vi "Apply Speed.vi"(8 "error in (no error)":errorcluster, 11 "Tool Funnel in":refnum<class "Tool Funnel.lvclass">) -> (0 "error out":errorcluster, 3 "Tool Funnel out":refnum<class "Tool Funnel.lvclass">)   [LabVIEW 2019, in "Tool Funnel.lvclass"]
uses:
  Tool Funnel.lvclass
  Settings/ObjectSettings/ObjectSettings.lvclass/ObjectSettings.ctl
  Settings/Funnel Settings/Funnel Settings.lvclass
  C:/Users/Albro/Documents/GitHub/AFM-Lithography/lvsrc/Classes/Settings/ObjectSettings/ObjectSettings.lvclass
  Settings/ObjectSettings/ObjectSettings.lvclass
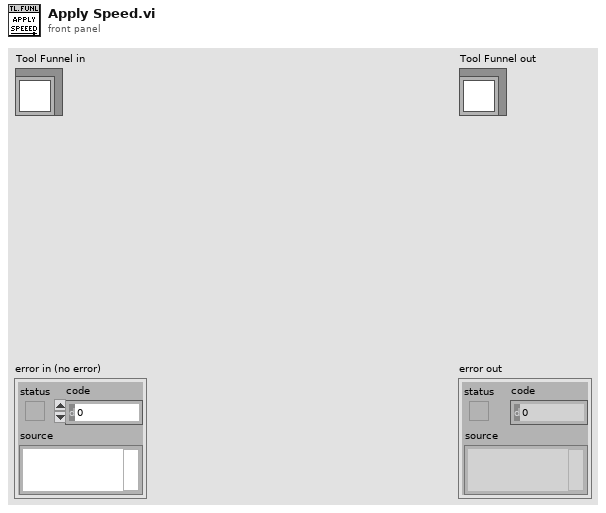
[diagram p1: front panel]
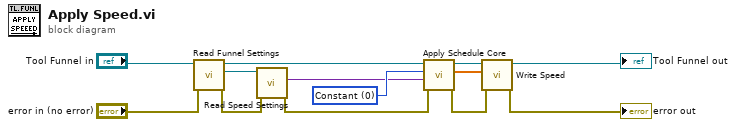
[diagram p0: block diagram]
diagram:
  w13 = u16 0 items=["Constant", "Ramp", "Function", "Formula"] ("Schedule")
  n1 = call-dynamic "Read Funnel Settings.vi"("error in (no error)"="error in (no error)", "Tool Funnel in"="Tool Funnel in") -> ("error out"=w2:errorcluster, "Funnel Settings.lvclass"=w3:refnum<class "Funnel Settings.lvclass">, "Tool Funnel out"=w4:refnum<class "Tool Funnel.lvclass">)  [unwired: 7 in]
  n2 = call "Read Speed Settings.vi"("error in (no error)"=w2, "ObjectSettings in"=w3) -> ("error out"=w9:errorcluster, "Settings"=w11:variant)  [unwired: 7 in, 1 out]
  n3 = call-dynamic "Apply Schedule Core.vi"("error in (no error)"=w9, "Settings"=w11, "Schedule"=w13, "Tool Object in"=w4) -> ("error out"=w10:errorcluster, "Schedule Array"=w8:dbl[], "Tool Object out"=w12:refnum<class "Tool Funnel.lvclass">)  [unwired: 5 in]
  n4 = call-dynamic "Write Speed.vi"("error in (no error)"=w10, "Speed"=w8, "Tool Object in"=w12) -> ("error out"=→"error out":errorcluster, "Tool Object out"=→"Tool Funnel out":refnum<class "Tool Funnel.lvclass">)  [unwired: 7 in]
